vi "PCRE Test 2.vi"(10 "Values Table":string="{\n \"{test}\": 1\n}", 11 "Expression In":string="$test == true || $b == false && $c == false") -> (0 "error out":errorcluster, 1 "Reverse Polish Notation Token Stack":cluster{string, string}[](array[cluster]), 4 "Total Time":dbl format="%.6fsec", 5 "Result":T2, 6 "Compile Time":dbl format="%.6fsec")   [LabVIEW 2014]
uses:
  src/core/expression/FTW-Expr-BooleanExpressionResult.ctl
  src/core/error/FTW-ERR-ThrowError.vi
  src/core/error/FTW-ERR-NoErrorConstant.vi
  src/core/error/FTW-ERR-CallChain.vi
  src/core/string/FTW-STR-ReplaceWhitespace.vi
  src/core/regex/FTW-Regex.lvclass
panel:
  out "Whole Match Begin":i32
  out "Submatches":i32[](array[numeric])
  out "Capture Groups":string[](array[string])
  out "ALL Tokens":T1(array[cluster]) {"?"."callout_id" format="Callout: %d"; "?"."subject_current_pos" format="Subj Pos: %d"; "?"."subject_start_match_pos" format="SubjectBegin: %d"; "?"."cap_top" format="CaptureTop: %d"; "?"."cap_last" format="CaptureLast: %d"; "?"."patt_pos" format="Pattern: %d"}
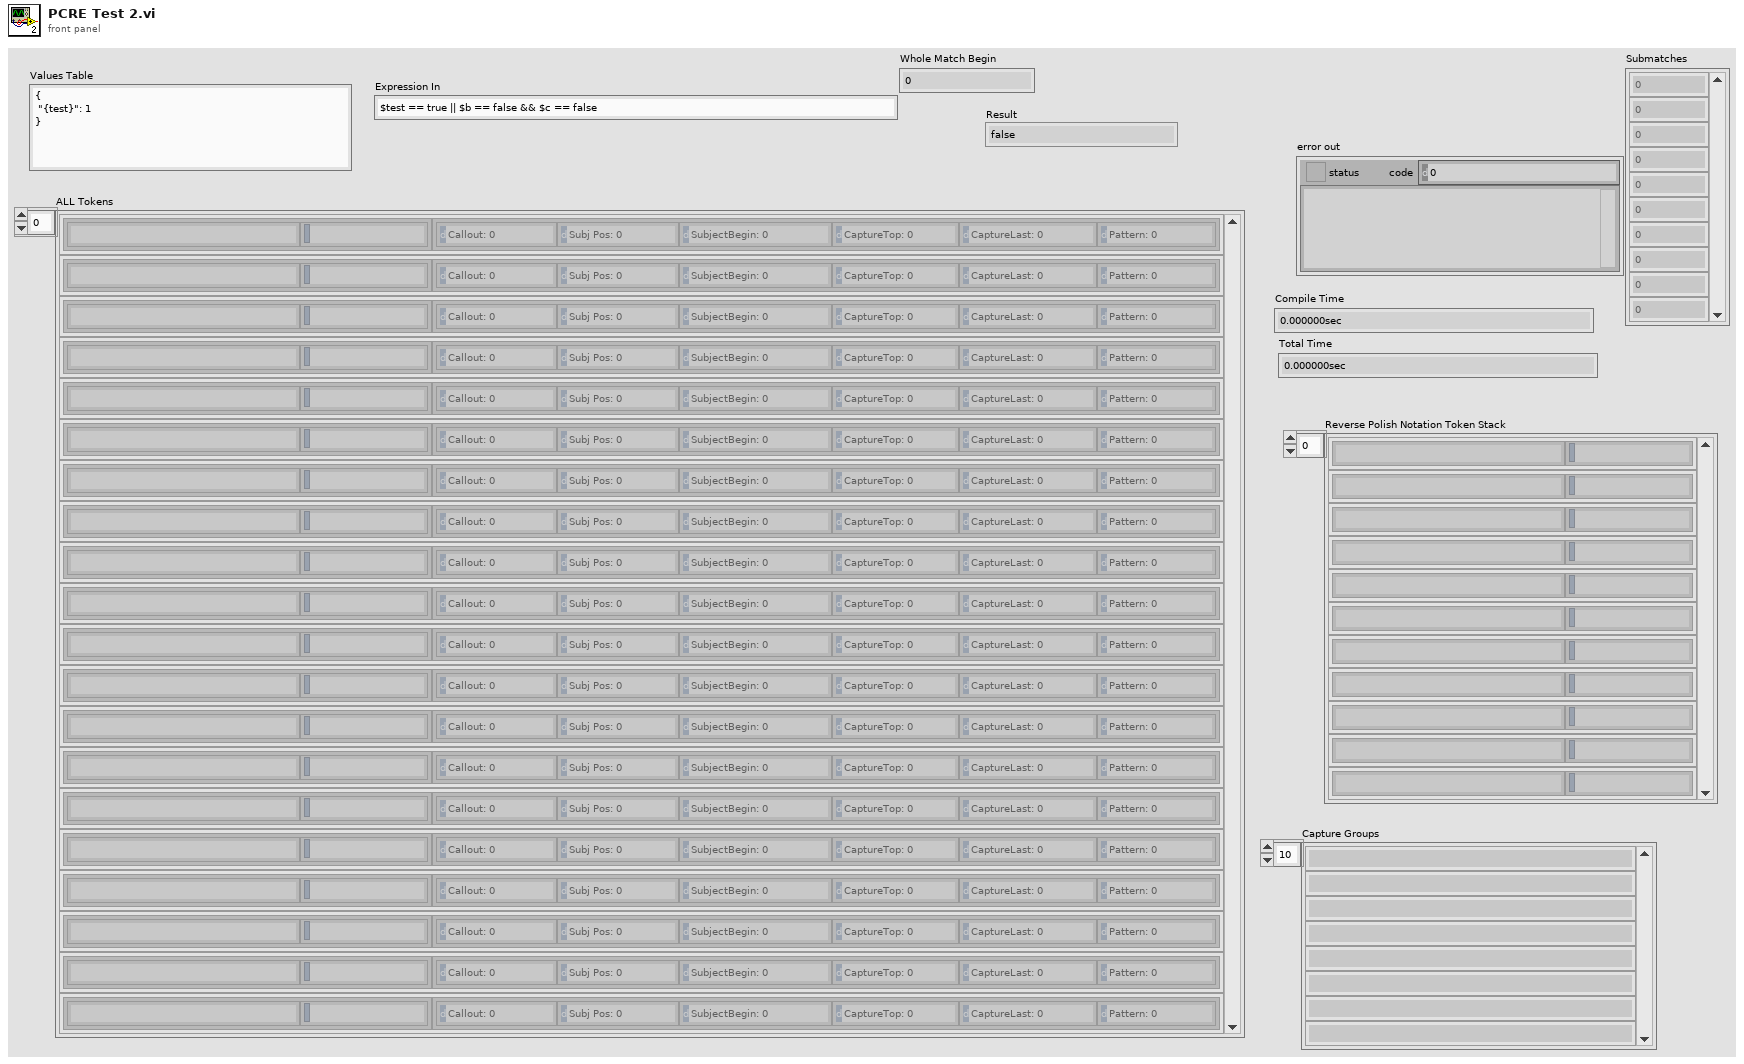
[diagram p1: front panel]
types:
  T1 = cluster{cluster{string, string}, cluster{"callout_id":i32, "subject_current_pos":i32, "subject_start_match_pos":i32, "cap_top":i32, "cap_last":i32, "patt_pos":i32}}[]
  T2 = typedef "FTW-Expr-BooleanExpressionResult.ctl" = enum16{"false", "true", "inconclusive"}
  T3 = cluster{"op":cluster{"token":string, "value":string}, "Precedence":i32, "Scope Depth":i32}[]
  T4 = cluster{"callout_id":i32, "subject_current_pos":i32, "subject_start_match_pos":i32, "cap_top":i32, "cap_last":i32, "patt_pos":i32}[]
  T5 = cluster{"callout_id":i32, "subject_current_pos":i32, "subject_start_match_pos":i32, "cap_top":i32, "cap_last":i32, "patt_pos":i32}
  T6 = cluster{cluster{string, "Expression In":string}, cluster{"callout_id":i32, "subject_current_pos":i32, "subject_start_match_pos":i32, "cap_top":i32, "cap_last":i32, "patt_pos":i32}}
  T7 = cluster{"token":string, "Expression In":string}[]
  T8 = cluster{cluster{string, "Expression In":string}, "Precedence":i32, i32}
  T9 = cluster{"op":cluster{"token":string, "value":string}, "Precedence":i32, "Scope Depth":i32}
  T10 = cluster{cluster{string, "Expression In":string}, "default value 1":i32, "Current Scope Depth":i32}
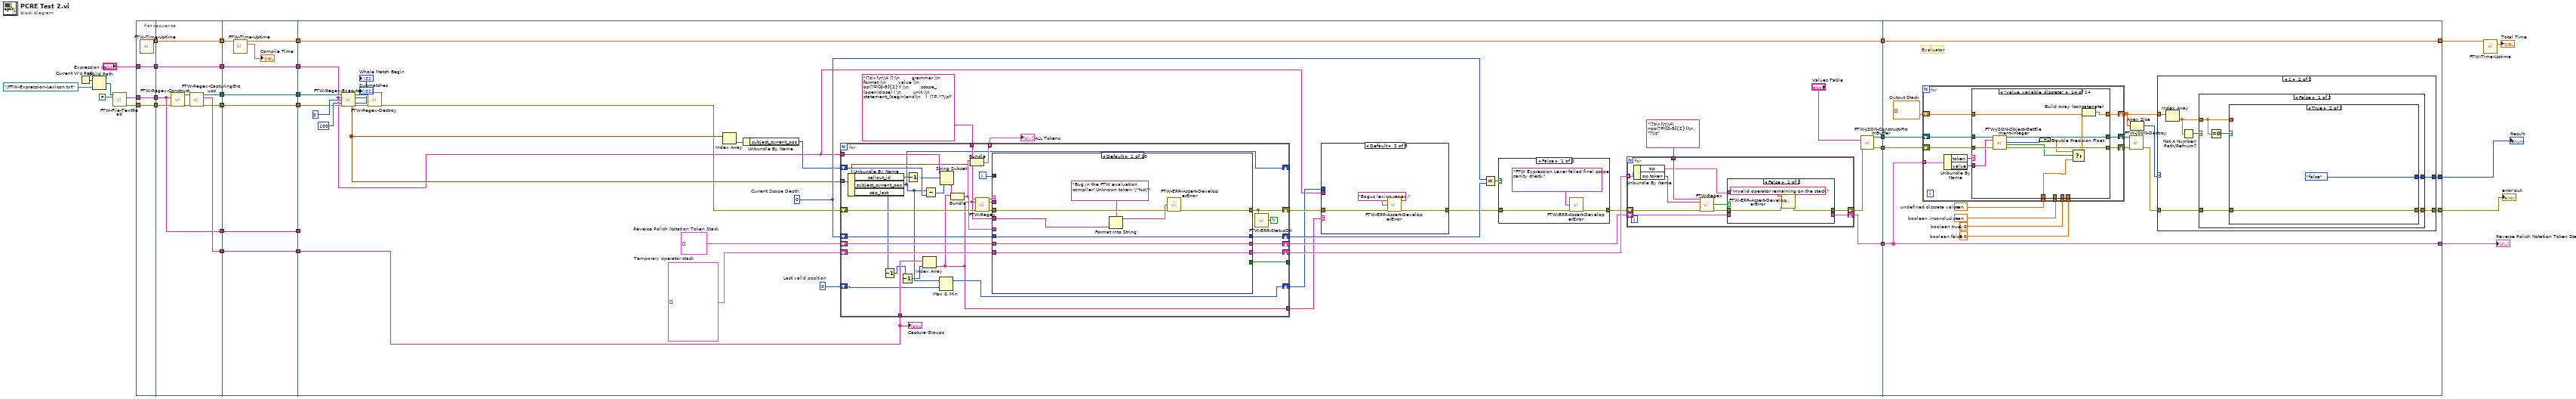
[diagram p0: block diagram]
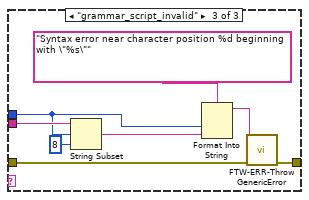
[diagram p3: hidden frame]
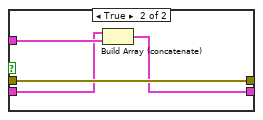
[diagram p5: hidden frame]
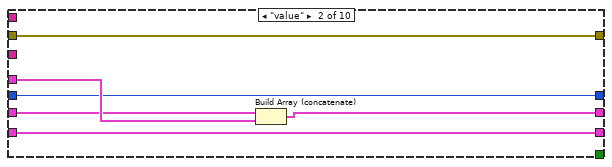
[diagram p6: hidden frame]
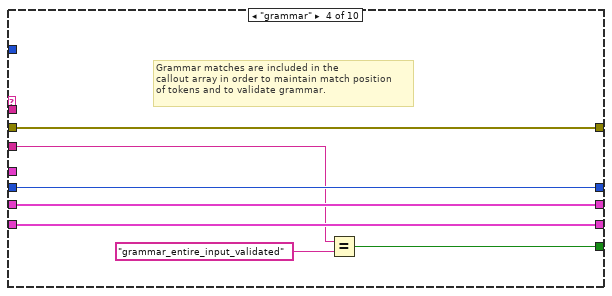
[diagram p8: hidden frame]
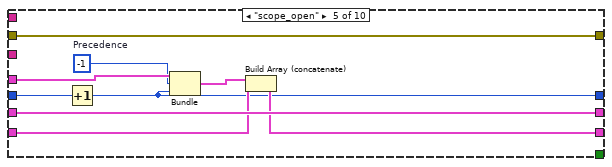
[diagram p9: hidden frame]
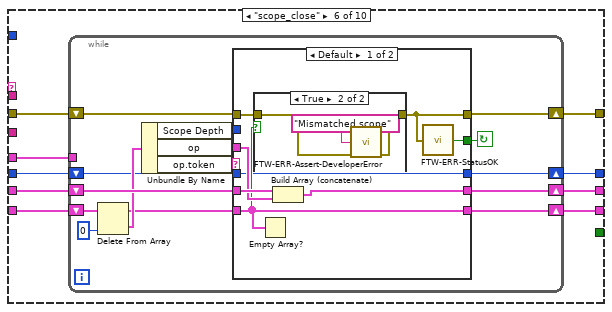
[diagram p10: hidden frame]
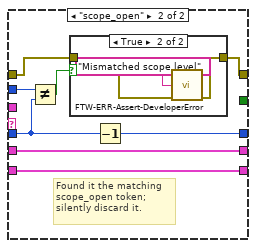
[diagram p12: hidden frame]
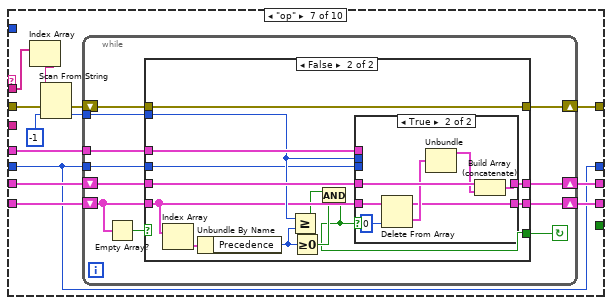
[diagram p14: hidden frame]
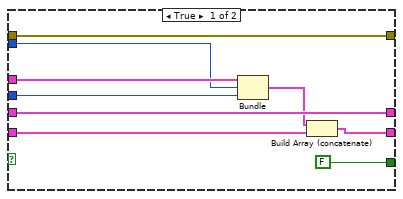
[diagram p15: hidden frame]
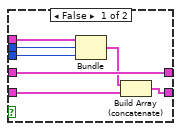
[diagram p16: hidden frame]
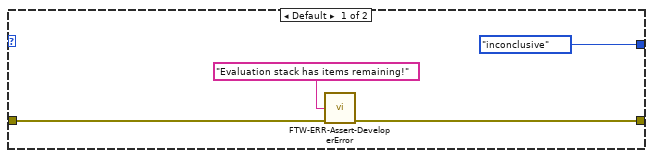
[diagram p20: hidden frame]
diagram:
  n1 = Current VI's Path() -> (path=w10:path)
  n2 = Build Path(base path=w10, name or relative path=path "../FTW-Expression-Lexicon.txt" ("path")) -> (appended path=w9:path)
  n3 = call "FTW-File-TextRead.vi"("Filepath"=w9, "Create if doesn't exist?"=FALSE) -> ("Text"=w32:string, "error out"=w3:errorcluster)  [unwired: 11 in, 1 out]
  n4 = flat-sequence {
    tunnel: w32 -> [w36]
    tunnel: [w36] -> w21
    tunnel: [w35] -> w19
    tunnel: [w34] -> w6
    tunnel: "Expression In" -> [w34]
    tunnel: [w33] -> w4
    tunnel: w3 -> [w33]
    tunnel: w21 -> [w37]
    tunnel: [w45] -> w20
    tunnel: w19 -> [w45]
    tunnel: [w42] -> w17
    tunnel: [w41] -> w15
    tunnel: [w40] -> w13
    tunnel: [w39] -> w7
    tunnel: w6 -> [w39]
    tunnel: w4 -> [w38]
    tunnel: [w37] -> w1
    tunnel: [w53] -> w28
    tunnel: w20 -> [w52]
    tunnel: [w51] -> w18
    tunnel: w17 -> [w51]
    tunnel: [w50] -> w16
    tunnel: w15 -> [w50]
    tunnel: [w49] -> w14
    tunnel: w13 -> [w49]
    tunnel: [w47] -> w8
    tunnel: w7 -> [w47]
    tunnel: [w46] -> w2
    tunnel: w1 -> [w46]
    tunnel: w28 -> [w82]
    tunnel: [w78] -> w26
    tunnel: [w83] -> w25
    tunnel: [w82] -> w24
    tunnel: [w81] -> w23
    tunnel: w18 -> [w69]
    tunnel: w16 -> [w65]
    tunnel: w14 -> [w68]
    tunnel: w8 -> [w57]
    tunnel: w2 -> [_]
    tunnel: [w324] -> w29
    tunnel: [w323] -> w30
    tunnel: [w315] -> w31
    tunnel: w26 -> [w320]
    tunnel: w25 -> [w323]
    tunnel: w24 -> [w324]
    tunnel: w23 -> [w321]
    tunnel: [w310] -> w22
    frame #0 {
      n5 = call "FTW-Time-Uptime.vi"() -> ("Current Uptime"=w35:dbl)  [unwired: 13 in, 2 out]
    }
    frame #1 {
      n6 = call "FTW-Regex-Construct.vi"("Regular Expression"=w37, "error in"=w38) -> ("Regex"=w43:refnum<class "FTW-Regex.lvclass">, "error out"=w44:errorcluster)  [unwired: 12 in]
      n7 = call "FTW-Regex-CapturingGroups.vi"("Regex"=w43, "error in"=w44) -> ("Regex out"=w42:refnum<class "FTW-Regex.lvclass">, "Capture Groups"=w41:string[], "error out"=w40:errorcluster)  [unwired: 11 in]
    }
    frame #2 {
      n8 = call "FTW-Time-Uptime.vi"("Previous Uptime"=w52) -> ("Current Uptime"=w53:dbl, "Elapsed Time"=→"Compile Time":dbl)  [unwired: 12 in, 1 out]
    }
    frame #3 {
      w59 = 0  # Last valid position
      w77 = 0  # Current Scope Depth
      w86 = T3 []  # Temporary operator stack
      w87 = cluster{"token":string, "value":string}[] []  # Reverse Polish Notation Token Stack
      n9 = call "FTW-Regex-Execute.vi"("Regex"=w69, "Subject String"=w57, "Starting Offset"=0, "Submatch Buffer Size"=100, "error in"=w68) -> ("Regex out"=w71:refnum<class "FTW-Regex.lvclass">, "Whole Match Begin"=→"Whole Match Begin":i32, "Submatches"=→"Submatches":i32[], "Callouts"=w66:T4, "error out"=w70:errorcluster)  [unwired: 5 in, 1 out]
      n10 = call "FTW-Regex-Destroy.vi"("Regex"=w71, "error in"=w70) -> ("error out"=w63:errorcluster)  [unwired: 13 in]
      n11 = Index Array(array=w66) -> (element=w89:T5)  [unwired: 1 in]
      n12 = Unbundle By Name(w89) -> ("subject_current_pos"=w67:i32)
      n13 = for {
        tunnel: "(?six)\n\\A (?:\n        grammar |\n        format |\n        value |\n        op(?=([0-9]{2})) |\n        scope_(open|close) | \n        unit |\n        statement_(begin|end)\n   )  (?=.*?\\z)" -> [w153]
        shift-right: [w149] -> w60
        shift-left: w87 -> [w150]
        shift-right: [w147] -> w62
        shift-left: w63 -> [w127]
        shift-right: [w145] -> w85
        shift-left: w86 -> [w144]
        shift-right: [w142] -> w76
        shift-left: w77 -> [w143]
        shift-right: [w130] -> _
        shift-left: w67 -> [w136]
        tunnel: w66 -> [w131] mode=indexing
        tunnel: w65 -> [w140]
        tunnel: w57 -> [w139]
        tunnel: [w132] -> w64 mode=indexing
        tunnel: [w134] -> _
        shift-right: [w128] -> w58
        shift-left: w59 -> [w129]
        tunnel: [w126] -> w56
        i -> [w135]
        stop <- w146 continue-if-true
        n14 = Unbundle By Name(w131) -> ("callout_id"=w141:i32, "subject_current_pos"=w130:i32, "cap_last"=w125:i32)
        n15 = Decrement(x=w125) -> (x-1=w124:i32)
        n16 = Decrement(x=w124) -> (x-1=w123:i32)
        n17 = Decrement(x=w141) -> ()  [unwired: 1 out]
        n18 = Index Array(array=w140, index=w123) -> (element=w126:string)
        n19 = Subtract(x=w130, y=w136) -> (x-y=w138:i32)
        n20 = Max & Min(x=w130, y=w129) -> (max(x,y)=w128:i32)  [unwired: 1 out]
        n21 = String Subset(string=w139, offset (0)=w136, length (rest)=w138) -> (substring=w137:string)
        n22 = Bundle(w126, "Expression In"=w137) -> (w133:cluster{string, "Expression In":string})  [unwired: 1 in]
        n23 = Bundle(w133, w131) -> (w132:T6)  [unwired: 1 in]
        n24 = call "FTW-Regex.vi"("Regular Expression"=w153, "Input String"=w126, "error in"=w127) -> ("Match"=w152:string, "Submatches"=w151:string[], "error out"=w148:errorcluster)  [unwired: 8 in, 2 out]
        n25 = case shown="Default" w152 {
          tunnel: w151 -> [_ _ _ _ _ _ w239 _ _ _]
          tunnel: w133 -> [_ w167 _ _ w183 w192 w240 _ _ _]
          tunnel: w150 -> [w159 w166 w171 w178 w186 w196 w244 w299 w303 w307]
          tunnel: [w159 w165 w171 w178 w186 w194 w245 w299 w303 w307] -> w149
          tunnel: [w160 w164 w170 w175 w187 w191 w242 w300 w304 w308] -> w147
          tunnel: w148 -> [w161 w164 w170 w175 w187 w190 w249 w300 w304 w308]
          tunnel: [w158 w163 w169 w177 w184 w193 w241 w298 w302 w306] -> w145
          tunnel: w144 -> [w158 w163 w169 w177 w185 w195 w246 w298 w302 w306]
          tunnel: w126 -> [w155 _ _ w174 _ _ _ _ _ _]
          tunnel: w143 -> [w154 w162 w168 w176 w181 w189 w237 w297 w301 w305]
          tunnel: [w154 w162 w168 w176 w180 w188 w237 w297 w301 w305] -> w142
          tunnel: w135 -> [_ _ _ _ _ _ _ _ _ _]
          tunnel: [_ _ _ w172 _ _ _ _ _ _] -> w134
          frame Default {
            n26 = Format Into String(format string="Bug in the FTW evaluation compiler! Unknown token: \"%s\"" ("Reason this error should never happen"), w155) -> (resulting string=w156:string)  [unwired: 2 in, 1 out]
            n27 = call "FTW-ERR-Assert-DeveloperError.vi"("Reason this error should never happen"=w156, "error in"=w161) -> ("error out"=w160:errorcluster)  [unwired: 13 in]
          }
          frame "value" {
            n28 = Build Array (concatenate)(w166, w167) -> (w165:T7)
          }
          frame "format" {
            # "Format matches are included in the\ncallout array purely to maintain match position\nof tokens."
          }
          frame "grammar" {
            # "Grammar matches are included in the\ncallout array in order to maintain match position\nof tokens and to validate grammar."
            n29 = Equal?(x=w174, y="grammar_entire_input_validated") -> (x = y?=w172:bool)
          }
          frame "scope_open" {
            w179 = -1  # Precedence
            n30 = Increment(x=w181) -> (x+1=w180:i32)
            n31 = Bundle(w183, "Precedence"=w179, w180) -> (w182:T8)  [unwired: 1 in]
            n32 = Build Array (concatenate)(w182, w185) -> (w184:T3)
          }
          frame "scope_close" {
            n33 = while {
              shift-right: [w202] -> w191
              shift-left: w190 -> [w203]
              shift-right: [w211] -> w194
              shift-left: w196 -> [w210]
              shift-right: [w209] -> w193
              shift-left: w195 -> [w208]
              tunnel: w192 -> [_]
              shift-right: [w199] -> w188
              shift-left: w189 -> [w198]
              stop <- w200 continue-if-true
              n34 = Delete From Array(array=w208, index=0) -> (deleted portion=w206:T9, array with subset deleted=w204:T3)  [unwired: 1 in]
              n35 = Unbundle By Name(w206) -> ("Scope Depth"=w197:i32, "op"=w201:cluster{"token":string, "value":string}, "op.token"=w205:string)
              n36 = case shown="Default" w205 {
                tunnel: [w220 w232] -> w211
                tunnel: w210 -> [w219 w232]
                tunnel: [w216 w231] -> w209
                tunnel: w204 -> [w216 w231]
                tunnel: w203 -> [w217 w227]
                tunnel: [w214 w226] -> w202
                tunnel: w201 -> [w218 _]
                tunnel: [w213 _] -> w200
                tunnel: [w212 w230] -> w199
                tunnel: w198 -> [w212 w228]
                tunnel: w197 -> [_ w229]
                frame Default {
                  n37 = Empty Array?(array=w216) -> (empty?=w215:bool)
                  n38 = case shown="True" w215 {
                    tunnel: w217 -> [w221 w224]
                    tunnel: [w221 w222] -> w214
                    frame False {
                    }
                    frame True {
                      n39 = call "FTW-ERR-Assert-DeveloperError.vi"("Reason this error should never happen"="Mismatched scope", "error in"=w224) -> ("error out"=w222:errorcluster)  [unwired: 13 in]
                    }
                  }
                  n40 = Build Array (concatenate)(w219, w218) -> (w220:cluster{"token":string, "value":string}[])
                  n41 = call "FTW-ERR-StatusOK.vi"("error to check"=w214) -> ("Status OK?"=w213:bool)
                }
                frame "scope_open" {
                  # "Found it the matching\nscope_open token;\nsilently discard it."
                  n42 = Not Equal?(x=w229, y=w228) -> (x != y?=w225:bool)
                  n43 = case shown="True" w225 {
                    tunnel: w227 -> [w233 w236]
                    tunnel: [w233 w234] -> w226
                    frame False {
                    }
                    frame True {
                      n44 = call "FTW-ERR-Assert-DeveloperError.vi"("Reason this error should never happen"="Mismatched scope level", "error in"=w236) -> ("error out"=w234:errorcluster)  [unwired: 13 in]
                    }
                  }
                  n45 = Decrement(x=w228) -> (x-1=w230:i32)
                }
              }
            }
          }
          frame "op" {
            n46 = Index Array(array=w239) -> (element=w238:string)  [unwired: 1 in]
            n47 = Scan From String(input string=w238, error in=w249, default 1=-1 ("default value 1")) -> (error out=w243:errorcluster, output 1=w247:i32)  [unwired: 2 in, 2 out]
            n48 = while {
              tunnel: w247 -> [w255]
              shift-right: [w251] -> w242
              shift-left: w243 -> [w250]
              shift-right: [w260] -> w245
              shift-left: w244 -> [w259]
              shift-right: [w258] -> w241
              shift-left: w246 -> [w257]
              tunnel: w240 -> [w256]
              tunnel: w237 -> [w254]
              stop <- w252 continue-if-true
              n49 = Empty Array?(array=w257) -> (empty?=w253:bool)
              n50 = case shown="False" w253 {
                tunnel: [w269 w282] -> w260
                tunnel: w259 -> [w269 w281]
                tunnel: [w268 w280] -> w258
                tunnel: w257 -> [w267 w276]
                tunnel: w256 -> [w266 w279]
                tunnel: w255 -> [w265 w278]
                tunnel: w254 -> [w264 w277]
                tunnel: [FALSE w270] -> w252
                tunnel: [w261 w274] -> w251
                tunnel: w250 -> [w261 w274]
                frame True {
                  n51 = Bundle(w266, "default value 1"=w265, "Current Scope Depth"=w264) -> (w263:T10)  [unwired: 1 in]
                  n52 = Build Array (concatenate)(w263, w267) -> (w268:T3)
                }
                frame False {
                  n53 = Index Array(array=w276) -> (element=w275:T9)  [unwired: 1 in]
                  n54 = Unbundle By Name(w275) -> ("Precedence"=w273:i32)
                  n55 = Greater Or Equal?(x=w278, y=w273) -> (x >= y?=w272:bool)
                  n56 = Greater Or Equal To 0?(x=w273) -> (x >= 0?=w271:bool)
                  n57 = And(x=w272, y=w271) -> (x .and. y?=w270:bool)
                  n58 = case shown="True" w270 {
                    tunnel: [w289 w295] -> w282
                    tunnel: w281 -> [w289 w296]
                    tunnel: [w287 w290] -> w280
                    tunnel: w276 -> [w288 w291]
                    tunnel: w279 -> [w286 _]
                    tunnel: w278 -> [w285 _]
                    tunnel: w277 -> [w283 _]
                    frame False {
                      n59 = Bundle(w286, "default value 1"=w285, "Current Scope Depth"=w283) -> (w284:T10)  [unwired: 1 in]
                      n60 = Build Array (concatenate)(w284, w288) -> (w287:T3)
                    }
                    frame True {
                      n61 = Delete From Array(array=w291, index=0) -> (deleted portion=w293:T9, array with subset deleted=w290:T3)  [unwired: 1 in]
                      n62 = Unbundle(w293) -> ("op"=w292:cluster{"token":string, "value":string})  [unwired: 2 out]
                      n63 = Build Array (concatenate)(w296, w292) -> (w295:cluster{"token":string, "value":string}[])
                    }
                  }
                }
              }
            }
          }
          frame "unit" {
          }
          frame "statement_begin" {
          }
          frame "statement_end" {
          }
        }
        n64 = call "FTW-ERR-StatusOK.vi"("error to check"=w147) -> ("Status OK?"=w146:bool)
      }
      "ALL Tokens" <- w64
      n65 = case shown="Default" w56 {
        tunnel: [w90 w92 w101] -> w61
        tunnel: w62 -> [w90 w93 w100]
        tunnel: w58 -> [_ _ w96]
        tunnel: w57 -> [_ _ w97]
        frame "grammar_script_valid" {
        }
        frame Default {
          n66 = call "FTW-ERR-Assert-DeveloperError.vi"("Reason this error should never happen"="Bogus lexing regex.", "error in"=w93) -> ("error out"=w92:errorcluster)  [unwired: 13 in]
        }
        frame "grammar_script_invalid" {
          n67 = String Subset(string=w97, offset (0)=w96, length (rest)=8 ("length (rest)")) -> (substring=w94:string)
          n68 = Format Into String(format string="Syntax error near character position %d beginning with \"%s\"" ("Error Message"), w96, w94) -> (resulting string=w98:string)  [unwired: 2 in, 1 out]
          n69 = call "FTW-ERR-ThrowGenericError.vi"("Error Message"=w98, "error in"=w100) -> ("error out"=w101:errorcluster)  [unwired: 13 in]
        }
      }
      n70 = Equal?(x=w77, y=w76) -> (x = y?=w75:bool)
      n71 = case shown="False" w75 {
        tunnel: w61 -> [w103 w105]
        tunnel: [w102 w105] -> w74
        frame False {
          n72 = call "FTW-ERR-Assert-DeveloperError.vi"("Reason this error should never happen"="FTW Expression Lexer failed final scope sanity check.", "error in"=w103) -> ("error out"=w102:errorcluster)  [unwired: 13 in]
        }
        frame True {
        }
      }
      n73 = for {
        tunnel: w85 -> [w115] mode=indexing
        shift-right: [w109] -> w79
        shift-left: w74 -> [w114]
        tunnel: "(?six)\n\\A\nop(?=([0-9]{2}))\n.*?\\z" ("Regular Expression") -> [w112]
        shift-right: [w106] -> w83
        shift-left: w60 -> [w107]
        n74 = Unbundle By Name(w115) -> ("op"=w108:cluster{"token":string, "value":string}, "op.token"=w113:string)
        n75 = call "FTW-Regex.vi"("Regular Expression"=w112, "Input String"=w113, "error in"=w114) -> ("Match Found?"=w111:bool, "error out"=w110:errorcluster)  [unwired: 8 in, 3 out]
        n76 = case shown="False" w111 {
          tunnel: w110 -> [w118 w122]
          tunnel: [w116 w122] -> w109
          tunnel: w108 -> [_ w121]
          tunnel: w107 -> [_ w120]
          tunnel: [_ w119] -> w106
          frame False {
            n77 = call "FTW-ERR-Assert-DeveloperError.vi"("Reason this error should never happen"="Invalid operator remaining on the stack.", "error in"=w118) -> ("error out"=w116:errorcluster)  [unwired: 13 in]
          }
          frame True {
            n78 = Build Array (concatenate)(w120, w121) -> (w119:cluster{"token":string, "value":string}[])
          }
        }
      }
      n79 = call "FTW-JSON-Construct-FromBuffer.vi"("JSON String (UTF-8)"="Values Table", "error in"=w79) -> ("JSON Object"=w81:refnum<data-value>, "error out"=w78:errorcluster)  [unwired: 12 in]
      "Capture Groups" <- w65
    }
    frame #4 {
      w309 = nan  # undefined discrete value
      w311 = nan  # boolean inconclusive
      w312 = 1.0  # boolean true
      w313 = 0.0  # boolean false
      w322 = dbl[] []  # Output Stack
      # "Evaluator"
      n80 = for {
        tunnel: w323 -> [w368] mode=indexing
        shift-right: [w365] -> w314
        shift-left: w322 -> [w366]
        shift-right: [w363] -> w319
        shift-left: w321 -> [w364]
        shift-right: [w361] -> w318
        shift-left: w320 -> [w362]
        tunnel: w313 -> [w359]
        tunnel: w312 -> [w358]
        tunnel: w311 -> [w357]
        tunnel: w309 -> [w356]
        n81 = Unbundle By Name(w368) -> ("token"=w367:string, "value"=w360:string)
        n82 = case shown="\"value_variable_discrete\"" w367 {
          selector: w367 -> [w370 _ _ _ _ _ _ _ _ _ _ _ _ _]
          tunnel: w366 -> [w376 w395 w414 w435 w456 w475 w489 w494 w499 w504 w509 w514 w524 w536]
          tunnel: [w376 w389 w408 w430 w451 w470 w487 w493 w497 w502 w508 w513 w523 w535] -> w365
          tunnel: w364 -> [w375 w388 w407 w429 w450 w469 w486 w492 w496 w501 w507 w512 w528 w540]
          tunnel: [w375 w388 w407 w429 w450 w469 w486 w492 w496 w501 w507 w512 w527 w539] -> w363
          tunnel: w362 -> [w374 w387 w406 w428 w449 w468 w485 w491 w495 w500 w506 w511 w526 w538]
          tunnel: [w373 w387 w406 w428 w449 w468 w485 w491 w495 w500 w506 w511 w525 w537] -> w361
          tunnel: w360 -> [w369 _ _ _ _ _ _ _ _ _ _ _ w522 w534]
          tunnel: w359 -> [_ w379 w398 w422 w443 w462 w478 _ _ _ w505 _ w517 _]
          tunnel: w358 -> [_ w378 w397 w417 w438 w460 w477 w490 _ _ _ _ w518 _]
          tunnel: w357 -> [_ w377 w396 w421 w442 w461 w483 _ _ _ _ w510 w519 _]
          tunnel: w356 -> [_ _ _ _ _ _ _ _ _ _ _ _ _ w532]
          frame Default {
            n83 = Format Into String(format string="Unhandled token '%s' with value '%s'" ("Reason this error should never happen"), w370, w369) -> (resulting string=w372:string)  [unwired: 2 in, 1 out]
            n84 = call "FTW-ERR-Assert-DeveloperError.vi"("Reason this error should never happen"=w372, "error in"=w374) -> ("error out"=w373:errorcluster)  [unwired: 13 in]
          }
          frame "op09_infix_discrete_equal" {
            n85 = Delete From Array(array=w395, index=0) -> (deleted portion=w385:dbl, array with subset deleted=w393:dbl[])  [unwired: 1 in]
            n86 = Delete From Array(array=w393, index=0) -> (deleted portion=w386:dbl, array with subset deleted=w390:dbl[])  [unwired: 1 in]
            n87 = Not A Number/Path/Refnum?(number/path/refnum=w385) -> (NaN/Path/Refnum?=w383:bool)
            n88 = Equal?(x=w386, y=w385) -> (x = y?=w391:bool)
            n89 = Not A Number/Path/Refnum?(number/path/refnum=w386) -> (NaN/Path/Refnum?=w384:bool)
            n90 = Or(x=w384, y=w383) -> (x .or. y?=w382:bool)
            n91 = Select(t=w378, s=w391, f=w379) -> (s? t:f=w381:dbl)
            n92 = Select(t=w377, s=w382, f=w381) -> (s? t:f=w380:dbl)
            n93 = Build Array (concatenate)(w380, w390) -> (w389:dbl[])
          }
          frame "op09_infix_discrete_noteql" {
            n94 = Delete From Array(array=w414, index=0) -> (deleted portion=w404:dbl, array with subset deleted=w412:dbl[])  [unwired: 1 in]
            n95 = Delete From Array(array=w412, index=0) -> (deleted portion=w405:dbl, array with subset deleted=w409:dbl[])  [unwired: 1 in]
            n96 = Not A Number/Path/Refnum?(number/path/refnum=w404) -> (NaN/Path/Refnum?=w402:bool)
            n97 = Not Equal?(x=w405, y=w404) -> (x != y?=w410:bool)
            n98 = Not A Number/Path/Refnum?(number/path/refnum=w405) -> (NaN/Path/Refnum?=w403:bool)
            n99 = Or(x=w403, y=w402) -> (x .or. y?=w401:bool)
            n100 = Select(t=w397, s=w410, f=w398) -> (s? t:f=w400:dbl)
            n101 = Select(t=w396, s=w401, f=w400) -> (s? t:f=w399:dbl)
            n102 = Build Array (concatenate)(w399, w409) -> (w408:dbl[])
          }
          frame "op14_infix_boolexpr_or" {
            n103 = Delete From Array(array=w435, index=0) -> (deleted portion=w418:dbl, array with subset deleted=w433:dbl[])  [unwired: 1 in]
            n104 = Delete From Array(array=w433, index=0) -> (deleted portion=w419:dbl, array with subset deleted=w431:dbl[])  [unwired: 1 in]
            n105 = Equal?(x=w418, y=w417) -> (x = y?=w416:bool)
            n106 = Not A Number/Path/Refnum?(number/path/refnum=w418) -> (NaN/Path/Refnum?=w426:bool)
            n107 = Equal?(x=w419, y=w417) -> (x = y?=w415:bool)
            n108 = Not A Number/Path/Refnum?(number/path/refnum=w419) -> (NaN/Path/Refnum?=w427:bool)
            n109 = Or(x=w415, y=w416) -> (x .or. y?=w420:bool)
            n110 = And(x=w427, y=w426) -> (x .and. y?=w425:bool)
            n111 = Select(t=w417, s=w420, f=w422) -> (s? t:f=w424:dbl)
            n112 = Select(t=w421, s=w425, f=w424) -> (s? t:f=w423:dbl)
            n113 = Build Array (concatenate)(w423, w431) -> (w430:dbl[])
          }
          frame "op13_infix_boolexpr_and" {
            n114 = Delete From Array(array=w456, index=0) -> (deleted portion=w439:dbl, array with subset deleted=w454:dbl[])  [unwired: 1 in]
            n115 = Delete From Array(array=w454, index=0) -> (deleted portion=w440:dbl, array with subset deleted=w452:dbl[])  [unwired: 1 in]
            n116 = Equal?(x=w439, y=w438) -> (x = y?=w437:bool)
            n117 = Not A Number/Path/Refnum?(number/path/refnum=w439) -> (NaN/Path/Refnum?=w447:bool)
            n118 = Equal?(x=w440, y=w438) -> (x = y?=w436:bool)
            n119 = Not A Number/Path/Refnum?(number/path/refnum=w440) -> (NaN/Path/Refnum?=w448:bool)
            n120 = And(x=w436, y=w437) -> (x .and. y?=w441:bool)
            n121 = Or(x=w448, y=w447) -> (x .or. y?=w446:bool)
            n122 = Select(t=w438, s=w441, f=w443) -> (s? t:f=w445:dbl)
            n123 = Select(t=w442, s=w446, f=w445) -> (s? t:f=w444:dbl)
            n124 = Build Array (concatenate)(w444, w452) -> (w451:dbl[])
          }
          frame "op09_infix_boolexpr_xor" {
            n125 = Delete From Array(array=w475, index=0) -> (deleted portion=w458:dbl, array with subset deleted=w473:dbl[])  [unwired: 1 in]
            n126 = Not A Number/Path/Refnum?(number/path/refnum=w458) -> (NaN/Path/Refnum?=w466:bool)
            n127 = Delete From Array(array=w473, index=0) -> (deleted portion=w457:dbl, array with subset deleted=w471:dbl[])  [unwired: 1 in]
            n128 = Not A Number/Path/Refnum?(number/path/refnum=w457) -> (NaN/Path/Refnum?=w467:bool)
            n129 = Not Equal?(x=w457, y=w458) -> (x != y?=w459:bool)
            n130 = Or(x=w467, y=w466) -> (x .or. y?=w465:bool)
            n131 = Select(t=w460, s=w459, f=w462) -> (s? t:f=w464:dbl)
            n132 = Select(t=w461, s=w465, f=w464) -> (s? t:f=w463:dbl)
            n133 = Build Array (concatenate)(w463, w471) -> (w470:dbl[])
          }
          frame "op03_prefix_boolexpr_not" {
            n134 = Delete From Array(array=w489, index=0) -> (deleted portion=w480:dbl, array with subset deleted=w482:dbl[])  [unwired: 1 in]
            n135 = Not A Number/Path/Refnum?(number/path/refnum=w480) -> (NaN/Path/Refnum?=w481:bool)
            n136 = Equal?(x=w480, y=w477) -> (x = y?=w479:bool)
            n137 = Select(t=w478, s=w479, f=w477) -> (s? t:f=w476:dbl)
            n138 = Select(t=w483, s=w481, f=w476) -> (s? t:f=w484:dbl)
            n139 = Build Array (concatenate)(w484, w482) -> (w487:dbl[])
          }
          frame "value_const_boolexpr_true" {
            n140 = Build Array (concatenate)(w490, w494) -> (w493:dbl[])
          }
          frame "value_const_discrete1" {
            w498 = 1.0  # discrete 1
            n141 = Build Array (concatenate)(w498, w499) -> (w497:dbl[])
          }
          frame "value_const_discrete0" {
            w503 = 0.0  # discrete 0
            n142 = Build Array (concatenate)(w503, w504) -> (w502:dbl[])
          }
          frame "value_const_boolexpr_false" {
            n143 = Build Array (concatenate)(w505, w509) -> (w508:dbl[])
          }
          frame "value_const_undefined" {
            n144 = Build Array (concatenate)(w510, w514) -> (w513:dbl[])
          }
          frame "value_variable_boolexpr" {
            n145 = call "FTW-JSON-Object-GetElement-Bool.vi"("JSON Object"=w528, "Key"=w522, "error in"=w526) -> ("JSON Object out"=w527:refnum<data-value>, "Value"=w515:bool, "Found?"=w516:bool, "error out"=w525:errorcluster)  [unwired: 9 in]
            n146 = Select(t=w518, s=w515, f=w517) -> (s? t:f=w521:dbl)
            n147 = Select(t=w521, s=w516, f=w519) -> (s? t:f=w520:dbl)
            n148 = Build Array (concatenate)(w520, w524) -> (w523:dbl[])
          }
          frame "value_variable_discrete" {
            n149 = call "FTW-JSON-Object-GetElement-Integer.vi"("JSON Object"=w540, "Key"=w534, "error in"=w538) -> ("JSON Object out"=w539:refnum<data-value>, "Value"=w529:i32, "Found?"=w530:bool, "error out"=w537:errorcluster)  [unwired: 9 in]
            n150 = To Double Precision Float(number=w529) -> (double precision float=w531:dbl)
            n151 = Select(t=w531, s=w530, f=w532) -> (s? t:f=w533:dbl)
            n152 = Build Array (concatenate)(w533, w536) -> (w535:dbl[])
          }
        }
      }
      n153 = call "FTW-JSON-Destroy.vi"("JSON Object"=w319, "error in"=w318) -> ("error out"=w316:errorcluster)  [unwired: 13 in]
      n154 = Array Size(array=w314) -> (size(s)=w317:i32)
      n155 = case shown="1" w317 {
        tunnel: w316 -> [w328 w332]
        tunnel: [w327 w333] -> w315
        tunnel: w314 -> [_ w334]
        tunnel: [FTW-Expr-BooleanExpressionResult."inconclusive" ("Result") w330] -> w310
        frame Default {
          n156 = call "FTW-ERR-Assert-DeveloperError.vi"("Reason this error should never happen"="Evaluation stack has items remaining!", "error in"=w328) -> ("error out"=w327:errorcluster)  [unwired: 13 in]
        }
        frame 1 {
          n157 = Index Array(array=w334) -> (element=w329:dbl)  [unwired: 1 in]
          n158 = Not A Number/Path/Refnum?(number/path/refnum=w329) -> (NaN/Path/Refnum?=w331:bool)
          n159 = case shown="False" w331 {
            tunnel: [w339 w354] -> w333
            tunnel: w332 -> [w338 w354]
            tunnel: [w336 FTW-Expr-BooleanExpressionResult."inconclusive" ("Result")] -> w330
            tunnel: w329 -> [w335 _]
            frame False {
              n160 = Equal To 0?(x=w335) -> (x = 0?=w337:bool)
              n161 = case shown="True" w337 {
                tunnel: [w344 w353] -> w339
                tunnel: w338 -> [w345 w353]
                tunnel: [w340 FTW-Expr-BooleanExpressionResult."false" ("Result")] -> w336
                tunnel: w335 -> [w343 _]
                frame False {
                  n162 = Equal?(x=w343, y=1.0) -> (x = y?=w341:bool)
                  n163 = case shown="True" w341 {
                    tunnel: w345 -> [w348 w350]
                    tunnel: [w347 w350] -> w344
                    tunnel: [FTW-Expr-BooleanExpressionResult."inconclusive" ("Result") FTW-Expr-BooleanExpressionResult."true" ("Result")] -> w340
                    frame False {
                      n164 = call "FTW-ERR-Assert-DeveloperError.vi"("Reason this error should never happen"="Boolean expression evaluated to non-Boolean result!", "error in"=w348) -> ("error out"=w347:errorcluster)  [unwired: 13 in]
                    }
                    frame True {
                    }
                  }
                }
                frame True {
                }
              }
            }
            frame True {
            }
          }
        }
      }
    }
  }
  n165 = call "FTW-Time-Uptime.vi"("Previous Uptime"=w29) -> ("Elapsed Time"=→"Total Time":dbl)  [unwired: 12 in, 2 out]
  "error out" <- w31
  "Reverse Polish Notation Token Stack" <- w30
  "Result" <- w22
